vi "Test Card Simulator Button Remains Pressed.vi"(8 "error in (no error)":errorcluster, 11 "Test Case In":refnum<class "View Model Test.lvclass">) -> (0 "error out":errorcluster, 3 "Test Case Out":refnum<class "View Model Test.lvclass">)   [LabVIEW 2020, in "View Model Test.lvclass"]
uses:
  View Model Test.lvclass
  C:/Program Files (x86)/National Instruments/LabVIEW 2020/vi.lib/Astemes/LUnit/Test Case.lvclass
  ATM View Model/Controls.ctl
  ATM Controller/State.ctl
  <vilib>/Astemes/LUnit/Test Case.lvclass/Test Case.ctl
  <vilib>/Astemes/LUnit/Palette/Fail.vi
  <vilib>/Astemes/LUnit/Palette/Pass.vi
  <vilib>/Astemes/LUnit/Set Assertion Type.vi
  <vilib>/Astemes/LUnit/Add test result.vi
  <vilib>/Astemes/LUnit/LUnit Record Assertion Result.vi
  <vilib>/Astemes/LUnit/LUnit Aggregate Assertion Results.vi
  <vilib>/Astemes/LUnit/Method Result/LUnit Merge Status.vi
  <vilib>/Astemes/LUnit/LUnit Concatenate result strings.vi
  ATM View Model/ATM View Model.lvclass
  ATM Controller/ATM Controller.lvclass
  <vilib>/Astemes/LUnit/Test Case.lvclass
panel:
  in  "Test Control":bool=TRUE
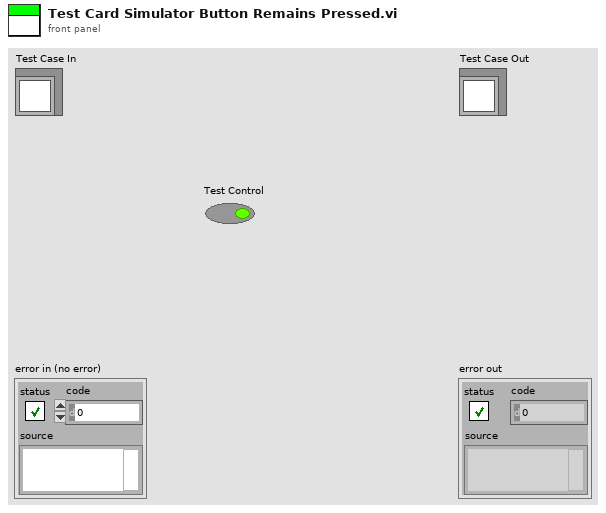
[diagram p1: front panel]
types:
  T1 = typedef "ATM Controller.lvclass/State.ctl" = enum16{"Start", "Insert Card", "Deposit", "Withdraw", "Fast Cash", "None", "Balance Inquiry", "Return Card"}
  T2 = typedef "ATM View Model.lvclass/Controls.ctl" = enum16{"User Input", "Enter", "Left Menu", "Righ Menu", "Left Button", "Right Button", "Card Simulator"}
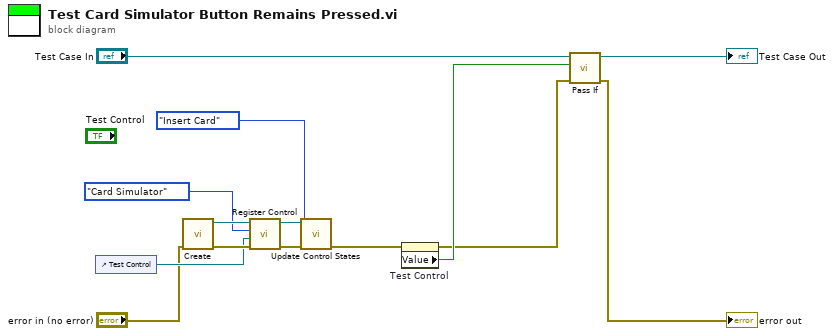
[diagram p0: block diagram]
diagram:
  n1 = control-ref of="Test Control"() -> (w7:refnum<vi>)
  n2 = call "Create.vi"("error in (no error)"="error in (no error)") -> ("error out"=w10:errorcluster, "ATM View Model out"=w11:refnum<class "ATM View Model.lvclass">)  [unwired: 9 in]
  n3 = call "Register Control.vi"("error in (no error)"=w10, "Control ref"=w7, "Control"=Controls."Card Simulator" ("Controls"), "ATM View Model in"=w11) -> ("error out"=w8:errorcluster, "ATM View Model out"=w9:refnum<class "ATM View Model.lvclass">)  [unwired: 6 in]
  n4 = call "Update Control States.vi"("error in (no error)"=w8, "ATM State"=State."Insert Card", "ATM View Model In"=w9) -> ("error out"=w5:errorcluster)  [unwired: 7 in, 1 out]
  n5 = property on="Test Control" class="Bool (strict)"(error in=w5) -> (error out=w2:errorcluster, "Value"=w4:bool)  [unwired: 1 in, 1 out]
  n6 = call <vilib>:"Pass If.vi"("error in (no error)"=w2, "Pass?"=w4, "LUnit Test Case In"="Test Case In") -> ("error out"=→"error out":errorcluster, "LUnit Test Case Out"=→"Test Case Out":refnum<class "View Model Test.lvclass">)  [unwired: 7 in]
